vi "Reset_Instr.vi"(8 "error in (no error)":errorcluster caption="entrée d'erreur (pas d'erreur)", 11 "Class Instrument (Default) en entrée":refnum<class "Class Instrument Printer.lvclass">) -> (0 "error out":errorcluster caption="sortie d'erreur", 3 "Class Instrument (Default) en sortie":refnum<class "Class Instrument Printer.lvclass">)   [LabVIEW 2020, in "Library Instrument & Equipement.lvlib" / "Library Instruments.lvlib" / "Class Instrument Printer.lvclass"]
uses:
  Class Instrument Printer.lvclass
  Instrument (Default)/Class Instrument (Default).lvclass
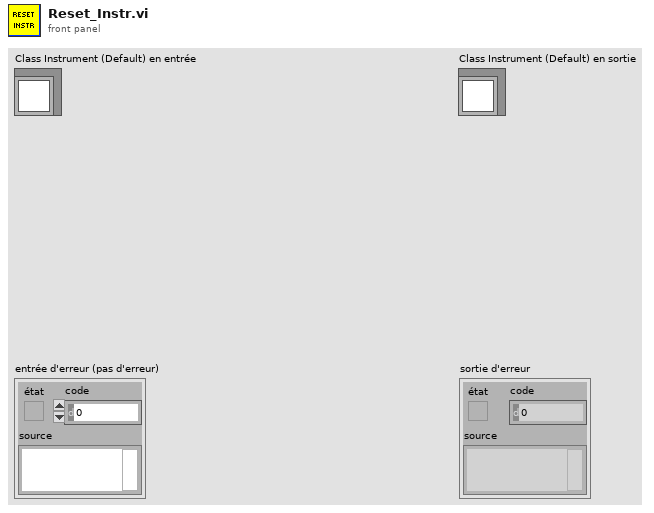
[diagram p1: front panel]
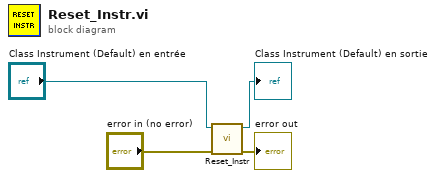
[diagram p0: block diagram]
diagram:
  n1 = call-parent "Reset_Instr.vi"("error in (no error)"="error in (no error)", "Class Instrument (Default) en entrée"="Class Instrument (Default) en entrée") -> ("error out"=→"error out":errorcluster, "Class Instrument (Default) en sortie"=→"Class Instrument (Default) en sortie":refnum<class "Class Instrument Printer.lvclass">)  [unwired: 8 in]
